vi "PlanckExperiment_LegacyMain_Copy.vi"() -> ()   [LabVIEW 2015]
uses:
  <vilib>/Instr/_visa.llb/VISA Configure Serial Port (Instr).vi
panel:
  out "串口状态灯":bool
  in  "发送":string
  out "接收":string
  in  "flow control (0:none)":u16(ring) caption="流控制（0:无）" items=["无", "XON/XOFF", "RTS/CTS", "XON/XOFF & RTS/CTS", "DTR/DSR", "XON/XOFF & DTR/DSR"]
  in  "stop bits (10: 1 bit)":u16=10 caption="停止位（10: 1位）"
  in  "波特率(默认9600)":u32=9600
  in  "停止":bool
  in  "发送":bool
  in  "奇偶 (0:none)":enum16{"None", "Odd", "Even", "Mark", "Space"}(ring) caption="奇偶（0:无）"
  in  "数据比特(默认8)":u16(ring)=8 items=["5"=5, "6"=6, "7"=7, "8"=8]
  in  "端口":refnum<visa-resource-name>="COM1"
  # "串口调试助手状态机\n三部分组成：\n1、状态机本身（枚举）\n①界面初始化\n②打开串口\n③等待用户触发（读取、写入）\n④关闭串口\n⑤退出\n2、选择分支\n3、While循环结构（重点移位寄存器）"
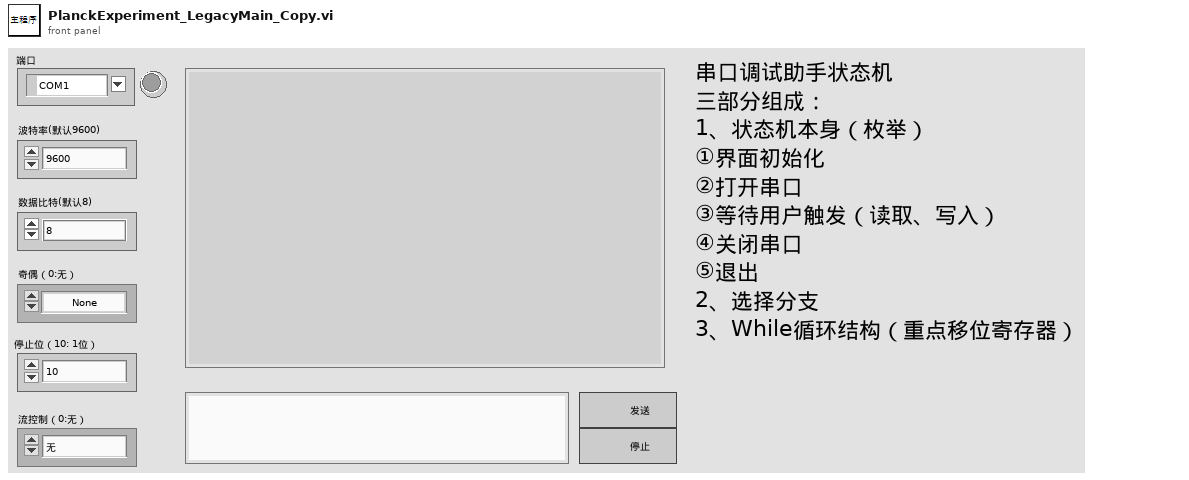
[diagram p1: front panel]
types:
  T1 = typedef "状态机0.ctl" = enum16{"初始化", "打开串口", "等待用户触发", "读取", "写入", "关闭串口", "退出"}
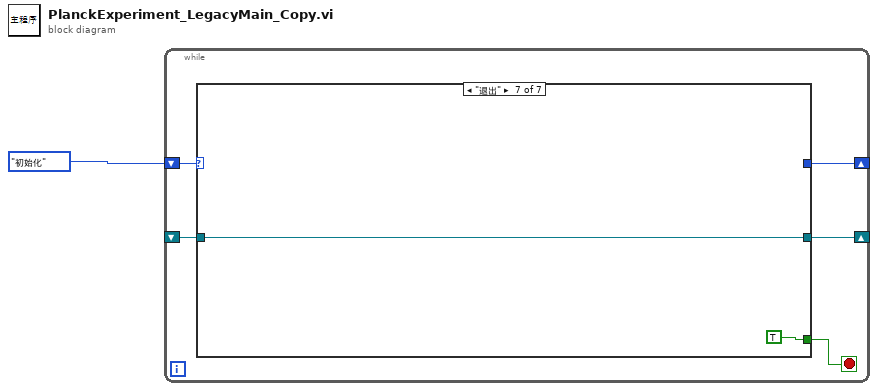
[diagram p0: block diagram]
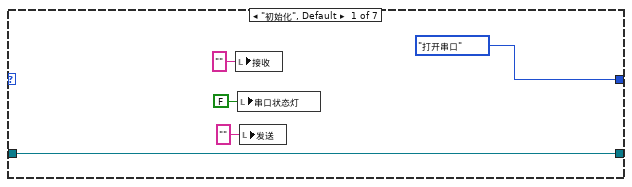
[diagram p2: hidden frame]
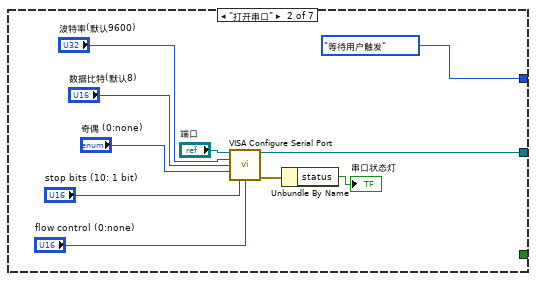
[diagram p3: hidden frame]
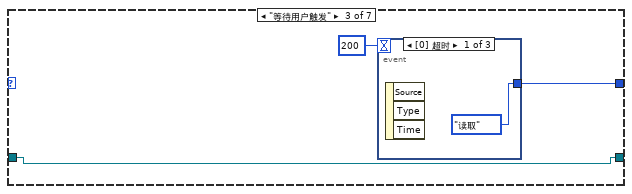
[diagram p4: hidden frame]
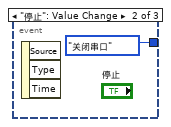
[diagram p5: hidden frame]
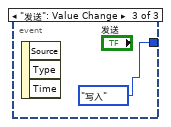
[diagram p6: hidden frame]
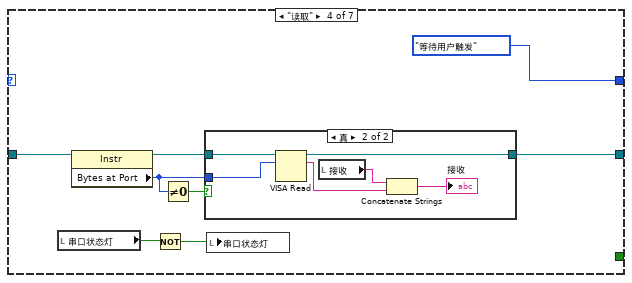
[diagram p7: hidden frame]
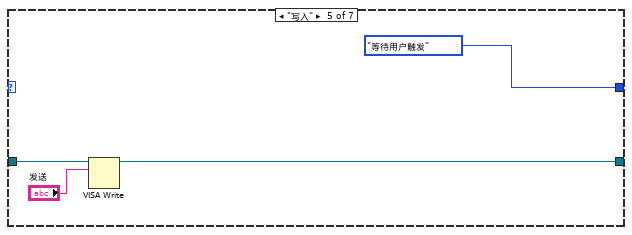
[diagram p9: hidden frame]
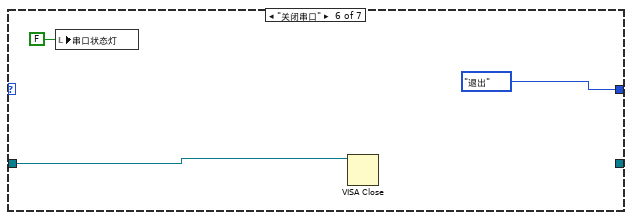
[diagram p10: hidden frame]
diagram:
  n1 = while {
    shift-right: [w5] -> _
    shift-left: 状态机0."初始化" ("状态机") -> [w6]
    shift-right: [w3] -> _
    shift-left: _ -> [w2]
    stop <- w4 stop-if-true
    n2 = case shown="\"退出\"" w6 {
      tunnel: [状态机0."打开串口" ("状态机") 状态机0."等待用户触发" ("状态机") w24 状态机0."等待用户触发" ("状态机") 状态机0."等待用户触发" ("状态机") 状态机0."退出" ("状态机") _] -> w5
      tunnel: [_ _ _ _ _ _ TRUE] -> w4
      tunnel: [w11 w15 w22 w35 w45 _ w50] -> w3
      tunnel: w2 -> [w11 _ w22 w34 w46 w48 w50]
      frame "初始化", Default {
        n3 = local write "接收"("" ("接收")) -> ()
        n4 = local write "串口状态灯"(FALSE ("串口状态灯")) -> ()
        n5 = local write "发送"("" ("发送")) -> ()
      }
      frame "打开串口" {
        n6 = call-poly "VISA Configure Serial Port"("VISA resource name"="端口", "baud rate (9600)"="波特率(默认9600)", "data bits (8)"="数据比特(默认8)", "parity (0:none)"="奇偶 (0:none)", "stop bits (10: 1 bit)"="stop bits (10: 1 bit)", "flow control (0:none)"="flow control (0:none)") -> ("VISA resource name out"=w15:refnum<visa-resource-name>, "error out"=w14:errorcluster)  [unwired: 8 in]
        n7 = Unbundle By Name(w14) -> ("status"=→"串口状态灯":bool)
      }
      frame "等待用户触发" {
        n8 = event shown="[0] 超时" {
          selector: _ -> [_ _ _]
          dyn-events: _ -> [_ _ _]
          timeout: 200 -> [_ _ _]
          tunnel: [状态机0."读取" ("状态机") 状态机0."关闭串口" ("状态机") 状态机0."写入" ("状态机")] -> w24
          event Timeout {
            n9 = event-data() -> ()  [unwired: 1 in, 3 out]
          }
          event "停止": Value Change {
            n10 = event-data() -> ()  [unwired: 1 in, 3 out]
          }
          event "发送": Value Change {
            n11 = event-data() -> ()  [unwired: 1 in, 3 out]
          }
        }
      }
      frame "读取" {
        n12 = local read "串口状态灯"() -> (w30:bool)
        n13 = property class="Instr"(reference=w34) -> (reference out=w33:refnum<visa-resource-name>, "Bytes at Port"=w31:u32)  [unwired: 1 in, 1 out]
        n14 = Not(x=w30) -> (.not. x?=w29:bool)
        n15 = Not Equal To 0?(x=w31) -> (x != 0?=w32:bool)
        n16 = case shown="真" w32 {
          tunnel: [w36 w42] -> w35
          tunnel: w33 -> [w36 w41]
          tunnel: w31 -> [_ w40]
          frame False {
          }
          frame True {
            n17 = VISA Read(VISA resource name=w41, byte count=w40) -> (VISA resource name out=w42:refnum<visa-resource-name>, read buffer=w38:string)  [unwired: 1 in, 2 out]
            n18 = local read "接收"() -> (w39:string)
            n19 = Concatenate Strings(w39, w38) -> (→"接收":string)
          }
        }
        n20 = local write "串口状态灯"(w29) -> ()
      }
      frame "写入" {
        n21 = VISA Write(VISA resource name=w46, write buffer="发送") -> (VISA resource name out=w45:refnum<visa-resource-name>)  [unwired: 1 in, 2 out]
      }
      frame "关闭串口" {
        n22 = local write "串口状态灯"(FALSE ("串口状态灯")) -> ()
        n23 = VISA Close(VISA resource name=w48) -> ()  [unwired: 1 in, 1 out]
      }
      frame "退出" {
      }
    }
  }
